vi "求导.vi"() -> ()   [LabVIEW 2015]
uses:
  <vilib>/Analysis/NI_AALPro.lvlib
panel:
  out "波形图 3":dbl[](graph)
  out "波形图 2":dbl[](graph)
  out "波形图":dynamicdata(graph)
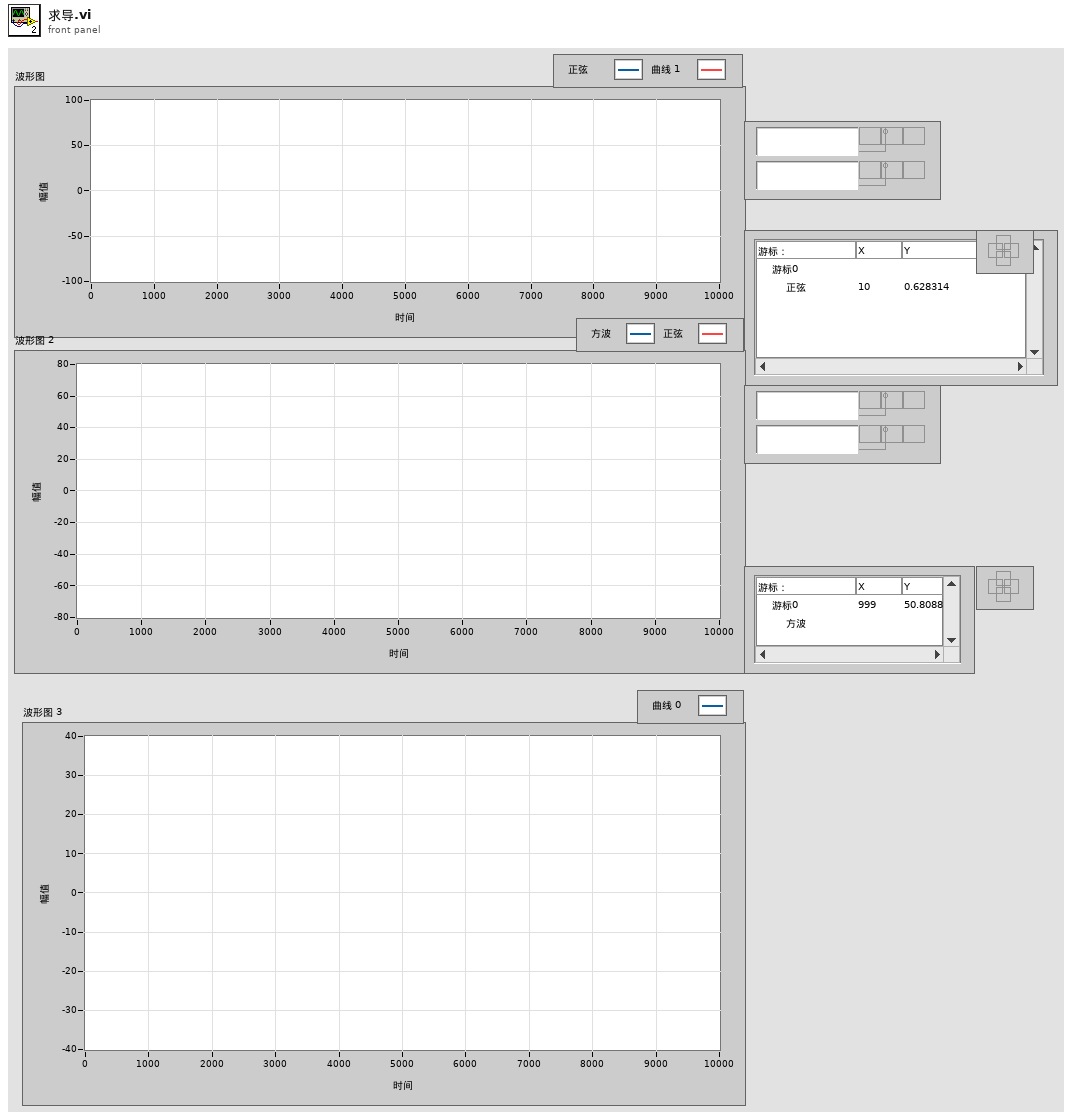
[diagram p1: front panel]
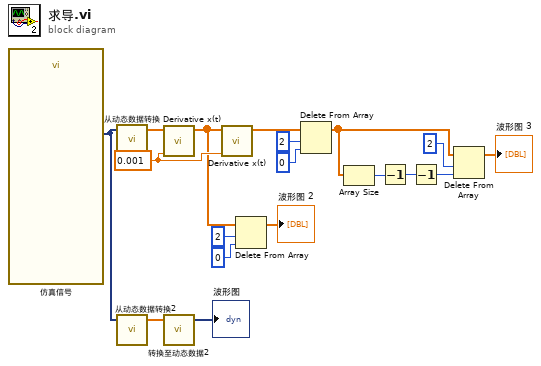
[diagram p0: block diagram]
diagram:
  w14 = 0.001 ("dt")
  n1 = call "仿真信号"() -> ("正弦"=w15:dynamicdata)  [unwired: 14 in, 1 out]
  n2 = call "从动态数据转换"("Dynamic Data Type"=w15) -> ("Array"=w16:dbl[])  [unwired: 3 in]
  n3 = call "从动态数据转换2"("Dynamic Data Type"=w15) -> ("Array"=w17:dbl[])  [unwired: 3 in]
  n4 = call <vilib>:"Derivative x(t).vi"("dt"=w14, "X"=w16) -> ("dX/dt"=w13:dbl[])  [unwired: 8 in, 1 out]
  n5 = call "转换至动态数据2"("Array"=w17) -> ("Dynamic Data Type"=→"波形图":dynamicdata)  [unwired: 3 in]
  n6 = call <vilib>:"Derivative x(t).vi"("dt"=w14, "X"=w13) -> ("dX/dt"=w7:dbl[])  [unwired: 8 in, 1 out]
  n7 = Delete From Array(array=w13, length=2 ("长度"), index=0 ("索引")) -> (array with subset deleted=→"波形图 2":dbl[])  [unwired: 1 out]
  n8 = Delete From Array(array=w7, length=2 ("长度"), index=0 ("索引")) -> (array with subset deleted=w4:dbl[])  [unwired: 1 out]
  n9 = Array Size(array=w4) -> (size(s)=w2:i32)
  n10 = Decrement(x=w2) -> (x-1=w3:i32)
  n11 = Decrement(x=w3) -> (x-1=w1:i32)
  n12 = Delete From Array(array=w4, length=2 ("长度"), index=w1) -> (array with subset deleted=→"波形图 3":dbl[])  [unwired: 1 out]
